vi "Handle Value Change.vi"(5 "VolatusAPI":refnum<class "VolatusAPI.lvclass">, 7 "CtlRef":refnum<vi>, 8 "error in (no error)":errorcluster, 9 "NewVal":variant, 10 "OldVal":variant, 11 "LoggingControl in":refnum<class "LoggingControl.lvclass">) -> (0 "error out":errorcluster, 3 "LoggingControl out":refnum<class "LoggingControl.lvclass">)   [LabVIEW 2020, in "VolatusGUIElements.lvlib" / "LoggingControl.lvclass"]
uses:
  LoggingControl.lvclass
  Volatus/VolatusAPI/VolatusAPI.lvclass
  LoggingControl.lvclass/LoggingControl.ctl
  Volatus/Event Level.ctl
  messages/StopLog/Data.ctl
  messages/StopLog/Class/Msg.lvclass/Msg.ctl
  Volatus/VolatusAPI/VolatusAPI.lvclass/VolatusAPI.ctl
  messages/StopLog/Class/Msg.lvclass
  C:/dev/lv20CE/relink/lv-protoc/LV-Proto/Message/Message.lvclass
  lv-vecto/Vecto/TCPMessageService/Send Message.vi
  <vilib>/Utility/error.llb/Error Cluster From Error Code.vi
  Log Prompt Async.vi
  lv-protoc/LV-Proto/Message/Message.lvclass
  Volatus/Volatus.lvlib
  messages/StopLog/StopLog.lvlib
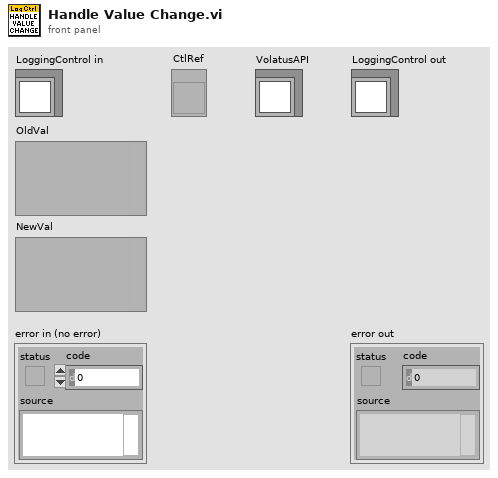
[diagram p1: front panel]
types:
  T1 = typedef "Volatus.lvlib/Event Level.ctl" = enum16{"Debug", "Info", "Warning", "Error"}
  T2 = enum8{"Enabled", "Disabled", "Disabled and Grayed Out"}
  T3 = typedef "StopLog.lvlib/Data.ctl" = cluster{"reason":string, "groups":string[]}
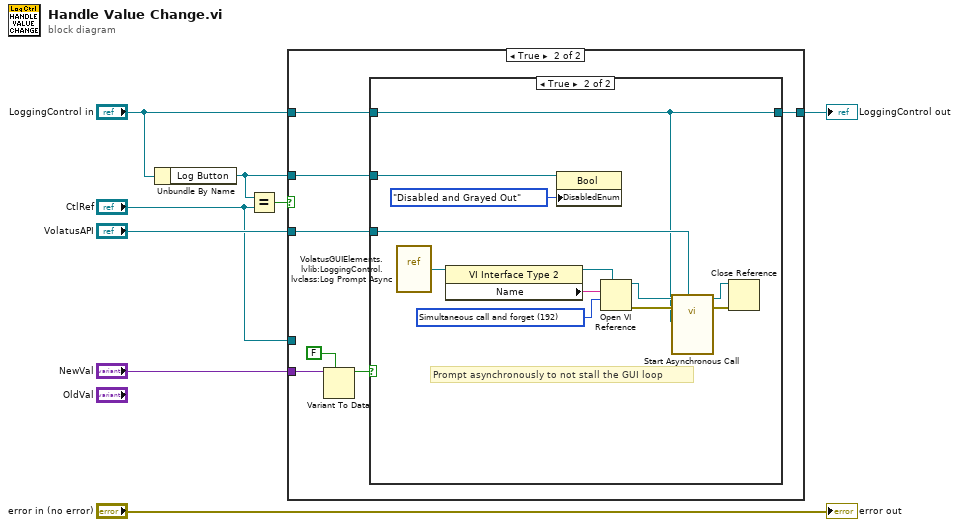
[diagram p0: block diagram]
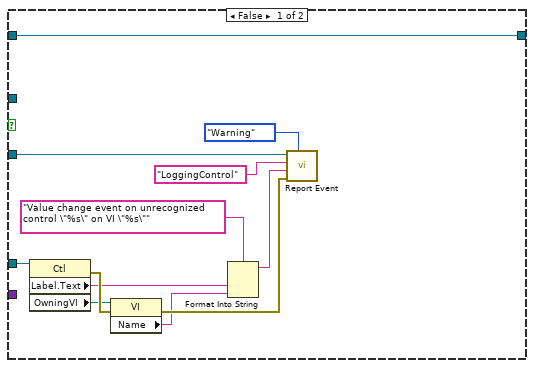
[diagram p2: hidden frame]
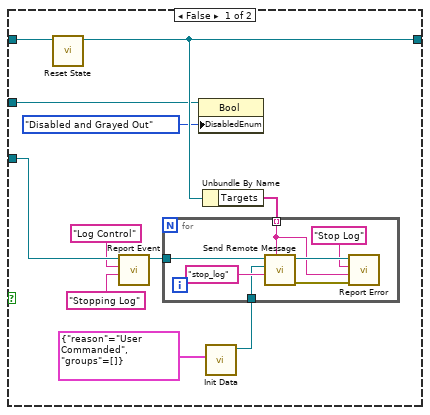
[diagram p3: hidden frame]
diagram:
  n1 = Unbundle By Name("LoggingControl in") -> ("Log Button"=w3:refnum<vi>)
  n2 = Equal?(x=w3, y="CtlRef") -> (x = y?=w6:bool)
  n3 = case shown="True" w6 {
    tunnel: "NewVal" -> [_ w27]
    tunnel: "VolatusAPI" -> [w18 w25]
    tunnel: "CtlRef" -> [w15 _]
    tunnel: w3 -> [_ w21]
    tunnel: "LoggingControl in" -> [w9 w24]
    tunnel: [w9 w22] -> w1
    frame False {
      n4 = property class="Ctl"(reference=w15) -> (error out=w19:errorcluster, "Label.Text"=w12:string, "OwningVI"=w14:refnum<vi>)  [unwired: 1 in, 1 out]
      n5 = property class="VI"(reference=w14, error in=w19) -> (error out=w20:errorcluster, "Name"=w11:string)  [unwired: 1 out]
      n6 = Format Into String(format string="Value change event on unrecognized control \"%s\" on VI \"%s\"", w12, w11) -> (resulting string=w10:string)  [unwired: 2 in, 1 out]
      n7 = call "Report Event.vi"("Level (Info)"=Event_Level."Warning", "error in (no error)"=w20, "Message"=w10, "Context"="LoggingControl", "VolatusAPI in"=w18) -> ()  [unwired: 5 in, 2 out]
    }
    frame True {
      n8 = Variant To Data(type=FALSE, Variant=w27) -> (data=w23:bool)  [unwired: 1 in, 1 out]
      n9 = case shown="True" w23 {
        tunnel: w25 -> [w38 w49]
        tunnel: w24 -> [w34 w48]
        tunnel: [w33 w48] -> w22
        tunnel: w21 -> [w31 w47]
        frame False {
          n10 = call "Reset State.vi"("LoggingControl in"=w34) -> ("LoggingControl out"=w33:refnum<class "LoggingControl.lvclass">)  [unwired: 9 in, 1 out]
          n11 = call "Report Event.vi"("Message"="Stopping Log" ("Context"), "Context"="Log Control", "VolatusAPI in"=w38) -> ("VolatusAPI out"=w30:refnum<class "VolatusAPI.lvclass">)  [unwired: 7 in, 1 out]
          n12 = property class="Bool"(reference=w31, "DisabledEnum"=T2."Disabled and Grayed Out" ("Disabled")) -> ()  [unwired: 1 in, 2 out]
          n13 = Unbundle By Name(w33) -> ("Targets"=w35:string[])
          n14 = call "Init Data.vi"("Data"=T3 {"reason"="User Commanded", "groups"=[]}) -> ("Msg out"=w36:refnum<class "Msg.lvclass">)  [unwired: 10 in]
          n15 = for {
            tunnel: w30 -> [w45]
            tunnel: w35 -> [w40] mode=indexing
            tunnel: w36 -> [w39]
            n16 = call "Send Remote Message.vi"("Target Name"=w40, "Message Type"="stop_log", "Message"=w39, "VolatusAPI in"=w45) -> ("error out"=w41:errorcluster, "VolatusAPI out"=w44:refnum<class "VolatusAPI.lvclass">)  [unwired: 6 in]
            n17 = call "Report Error.vi"("error in (no error)"=w41, "Message"=w40, "Context"="Stop Log", "VolatusAPI in"=w44) -> ()  [unwired: 6 in, 2 out]
          }
        }
        frame True {
          w52 = 192 items=["Record modifications"=1, "Open templates for editing"=2, "Prompt user to save"=4, "Prepare for reentrant run"=8, "Prompt to find missing subVIs"=16, "Hide loading dialog box"=32, "Enable simultaneous calls"=64, "Prepare to call and forget"=128, "Simultaneous call and forget"=192, "Prepare to call and collect"=256, "Simultaneous call and collect"=320]
          # "Prompt asynchronously to not stall the GUI loop"
          n18 = vi-ref "VolatusGUIElements.lvlib:LoggingControl.lvclass:Log Prompt Async.vi"() -> (w50:refnum<vi>)
          n19 = property class="VI Interface Type 2"(reference=w50) -> (reference out=w53:refnum<vi>, "Name"=w51:string)  [unwired: 1 in, 1 out]
          n20 = property class="Bool"(reference=w47, "DisabledEnum"=T2."Disabled and Grayed Out" ("Disabled")) -> ()  [unwired: 1 in, 2 out]
          n21 = Open VI Reference(type specifier VI Refnum (for type only)=w53, vi path=w51, options=w52) -> (vi reference=w55:refnum<vi>, error out=w54:errorcluster)  [unwired: 3 in]
          n22 = call-by-ref "Start Asynchronous Call"(reference=w55, error in=w54, "VolatusAPI"=w49, "LoggingControl in"=w48) -> (reference out=w57:refnum<vi>, error out=w56:errorcluster)  [unwired: 10 in]
          n23 = Close Reference(reference=w57, error in (no error)=w56) -> ()  [unwired: 1 out]
        }
      }
    }
  }
  "LoggingControl out" <- w1
  "error out" <- "error in (no error)"
